vi "Format SQL INSERT.vi"(8 "error in":errorcluster, 9 "Time Stamp":timestamp, 10 "Data":variant, 11 "Path(s)":variant) -> (0 "error out":errorcluster, 2 "Formatted Insert":string)   [LabVIEW 2013, in "Data.PGSQL.lvclass"]
uses:
  Data.PGSQL.lvclass
  Typedefs/Errors--enum.ctl
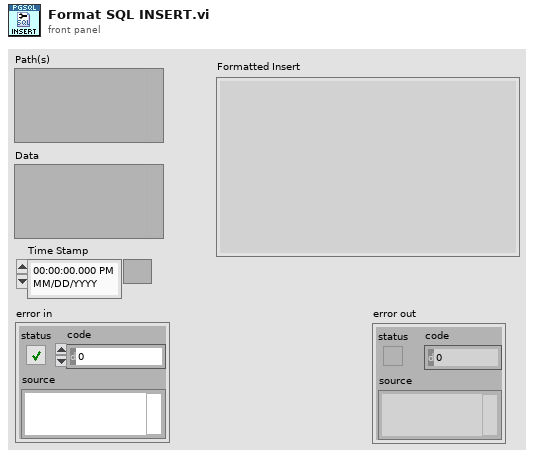
[diagram p1: front panel]
types:
  T1 = typedef "Data.PGSQL.lvclass/Errors--enum.ctl" = enum16{"0: None", "5005: Path Type Not Supported", "5006: Number of Variables", "5008: Cannot write two data points", "5030: Start and End Times Identical", "5031: Input is not wholly", "5033: Bad path or paths", "5040: Invalid Instrument Name", "5050: Column can only hold string", "5051 Column can only hold bool", "5052: Column can only hold double", "5053: Column can only hold int"}
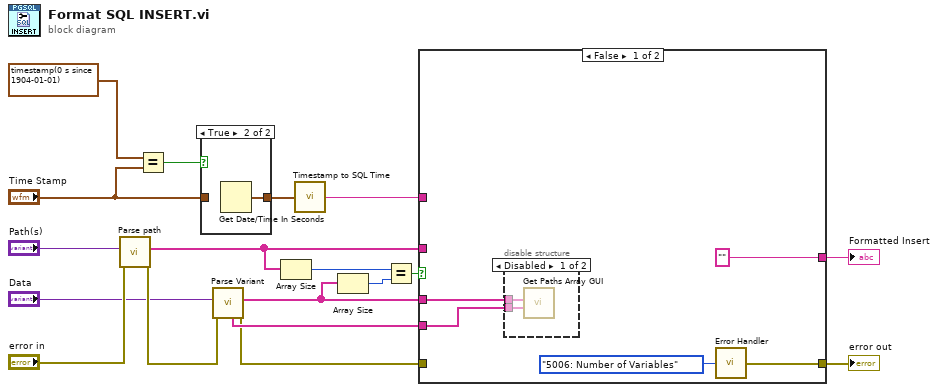
[diagram p0: block diagram]
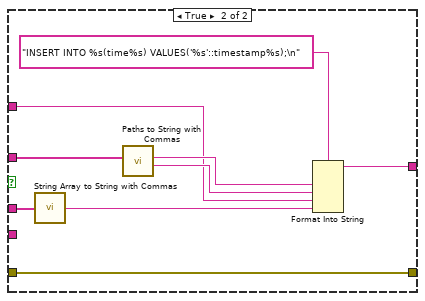
[diagram p3: hidden frame]
diagram:
  n1 = call "Parse path.vi"("error in"="error in", "Paths?"="Path(s)") -> ("error out"=w8:errorcluster, "Paths"=w2:string[])  [unwired: 8 in]
  n2 = Equal?(x=timestamp(0 s since 1904-01-01), y="Time Stamp") -> (x = y?=w18:bool)
  n3 = case shown="True" w18 {
    tunnel: [w19 w20] -> w7
    tunnel: "Time Stamp" -> [w19 _]
    frame False {
    }
    frame True {
      n4 = Get Date/Time In Seconds() -> (seconds since 1Jan1904=w20:timestamp)
    }
  }
  n5 = call "Parse Variant.vi"("error in"=w8, "variant"="Data") -> ("error out"=w3:errorcluster, "Strings"=w13:string[], "Types (strings)"=w5:string[])  [unwired: 5 in, 2 out]
  n6 = Array Size(array=w2) -> (size(s)=w16:i32)
  n7 = call "Timestamp to SQL Time.vi"("seconds since 1Jan1904"=w7) -> ("date/time string"=w6:string)
  n8 = Array Size(array=w13) -> (size(s)=w15:i32)
  n9 = Equal?(x=w16, y=w15) -> (x = y?=w14:bool)
  n10 = case shown="False" w14 {
    tunnel: w13 -> [w25 w36]
    tunnel: w2 -> [_ w35]
    tunnel: [w22 w29] -> w12
    tunnel: w3 -> [_ w29]
    tunnel: w6 -> [_ w31]
    tunnel: w5 -> [w23 _]
    tunnel: ["" w30] -> w10
    frame False {
      n11 = disable-structure shown="Disabled" {
        disable-tunnel: w25 -> [w27 _]
        disable-tunnel: w23 -> [w26 _]
        frame Disabled {
          n12 = call "Get Paths Array GUI.vi"("Types (string)"=w26, "Data"=w27) -> ()  [unwired: 10 in]
        }
        frame Enabled {
        }
      }
      n13 = call "Error Handler.vi"("Error code"=Errors--enum."5006: Number of Variables") -> ("error out"=w22:errorcluster)
    }
    frame True {
      n14 = call "String Array to String with Commas.vi"("Array"=w36) -> ("String"=w32:string)
      n15 = call "Paths to String with Commas.vi"("Array"=w35) -> ("Columns"=w33:string, "Table"=w34:string)  [unwired: 9 in]
      n16 = Format Into String(format string="INSERT INTO %s(time%s) VALUES('%s'::timestamp%s);\n", w34, w33, w31, w32) -> (resulting string=w30:string)  [unwired: 2 in, 1 out]
    }
  }
  "error out" <- w12
  "Formatted Insert" <- w10
